vi "pf_Get_Property_Data_Info.vi"(8 "error in (no error)":errorcluster, 10 "Property Name":string, 11 "IMAQ Session in":refnum<k11> caption="Camera Session in") -> (0 "error out":errorcluster, 1 "Property Data Info":T1, 2 "Property Name out":string, 3 "IMAQ Session out":refnum<k11> caption="Camera Session in")   [LabVIEW 2025, in "Photonfocus_Toolkit.lvlib"]
doc: "Gets information about the specified property."
uses:
  Photonfocus_Toolkit.lvlib
  _Private/Controls/pf_Property_Data_Info.ctl
  _Private/Controls/pf_Property_Type.ctl
  _Private/Controls/pf_Camera_ctrl_mngr_action.ctl
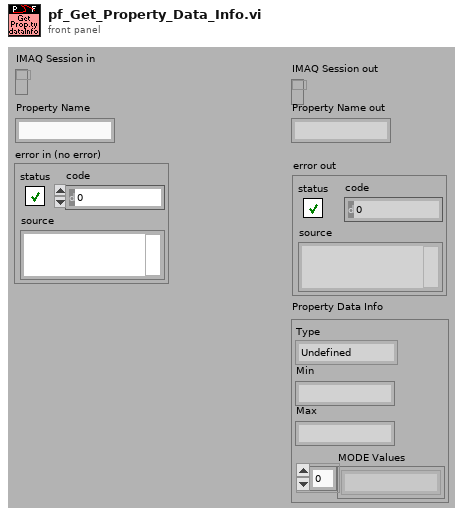
[diagram p1: front panel]
types:
  T1 = typedef "Photonfocus_Toolkit.lvlib/pf_Property_Data_Info.ctl" = cluster{"Type":T2, "Min":string, "Max":string, "MODE Values":string[]}
  T2 = typedef "Photonfocus_Toolkit.lvlib/pf_Property_Type.ctl" = enum16{"Undefined", "PF_ROOT", "PF_INT", "PF_FLOAT", "PF_BOOL", "PF_MODE", "PF_REGISTER", "PF_STRING", "PF_BUFFER", "PF_STRUCT", "PF_ARRAY", "PF_COMMAND", "PF_EVENT"}
  T3 = typedef "Photonfocus_Toolkit.lvlib/pf_Camera_ctrl_mngr_action.ctl" = enum16{"Create", "Destroy", "Set", "Get"}
  T4 = typedef "Photonfocus_Toolkit.lvlib/pf_Property_Cluster.ctl" = cluster{"Name":string, "Type":T2, "Float.Min":sgl, "Float.Max":sgl, "Float.Value":sgl, "Int.Min":u32, "Int.Max":u32, "Int.Value":u32, "String.Value":string, "MODE.Values":string[], "MODE.Index":i32, "Flag":T5}
  T5 = typedef "Photonfocus_Toolkit.lvlib/pf_Property_Flag.ctl" = enum16{"Undefined", "RO", "WO", "RW"}
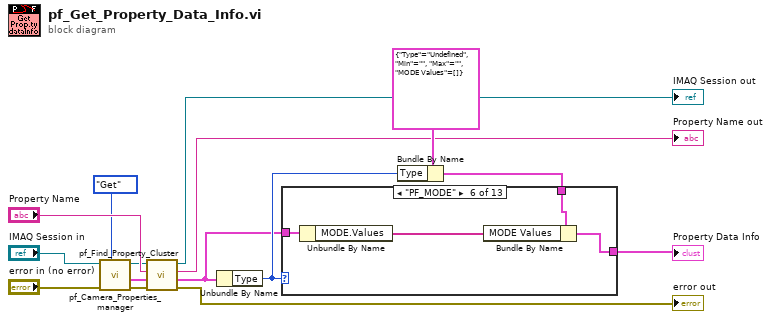
[diagram p0: block diagram]
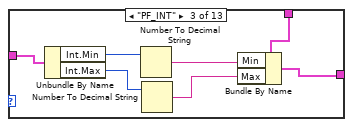
[diagram p4: hidden frame]
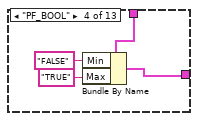
[diagram p5: hidden frame]
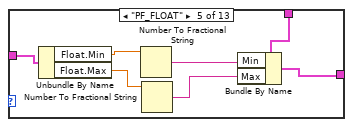
[diagram p6: hidden frame]
diagram:
  n1 = call "pf_Camera_Properties_manager.vi"("Action"=pf_Camera_ctrl_mngr_action."Get", "error in (no error)"="error in (no error)", "IMAQ Session in"="IMAQ Session in") -> ("error out"=w15:errorcluster, "Properties Array out"=w14:T4[], "IMAQ Session out"=w9:refnum<k11>)  [unwired: 1 in, 5 out]
  n2 = call "pf_Find_Property_Cluster.vi"("error in (no error)"=w15, "Properties Array"=w14, "Property Name"="Property Name", "IMAQ Session in"=w9) -> ("error out"=→"error out":errorcluster, "Property element"=w4:T4, "Property Name out"=→"Property Name out":string, "IMAQ Session out"=→"IMAQ Session out":refnum<k11>)  [unwired: 4 out]
  n3 = Unbundle By Name(w4) -> ("Type"=w7:T2)
  n4 = Bundle By Name(cluster=T1 {"Type"=enum."Undefined", "Min"="", "Max"="", "MODE Values"=[]} ("Property Value Info"), "Type"=w7) -> (w5:T1)
  n5 = case shown="\"PF_MODE\"" w7 {
    tunnel: [w16 w17 w18 w27 w29 w36 w40 w41 w42 w43 w44 w45 w46] -> w6
    tunnel: w5 -> [w16 w17 w21 w28 w32 w38 w40 w41 w42 w43 w44 w45 w46]
    tunnel: w4 -> [_ _ w24 _ w35 w39 _ _ _ _ _ _ _]
    frame "Undefined", Default {
    }
    frame "PF_ROOT" {
    }
    frame "PF_INT" {
      n6 = Unbundle By Name(w24) -> ("Int.Min"=w23:u32, "Int.Max"=w22:u32)
      n7 = Number To Decimal String(number=w23) -> (decimal integer string=w20:string)  [unwired: 1 out]
      n8 = Number To Decimal String(number=w22) -> (decimal integer string=w19:string)  [unwired: 1 out]
      n9 = Bundle By Name(cluster=w21, "Min"=w20, "Max"=w19) -> (w18:T1)
    }
    frame "PF_BOOL" {
      n10 = Bundle By Name(cluster=w28, "Min"="FALSE", "Max"="TRUE") -> (w27:T1)
    }
    frame "PF_FLOAT" {
      n11 = Unbundle By Name(w35) -> ("Float.Min"=w34:sgl, "Float.Max"=w33:sgl)
      n12 = Number To Fractional String(number=w34) -> (F-format string=w31:string)  [unwired: 3 out]
      n13 = Number To Fractional String(number=w33) -> (F-format string=w30:string)  [unwired: 3 out]
      n14 = Bundle By Name(cluster=w32, "Min"=w31, "Max"=w30) -> (w29:T1)
    }
    frame "PF_MODE" {
      n15 = Unbundle By Name(w39) -> ("MODE.Values"=w37:string[])
      n16 = Bundle By Name(cluster=w38, "MODE Values"=w37) -> (w36:T1)
    }
    frame "PF_REGISTER" {
    }
    frame "PF_STRING" {
    }
    frame "PF_BUFFER" {
    }
    frame "PF_STRUCT" {
    }
    frame "PF_ARRAY" {
    }
    frame "PF_COMMAND" {
    }
    frame "PF_EVENT" {
    }
  }
  "Property Data Info" <- w6
